vi "ReadFeatureList.vi"(8 "error in (no error)":errorcluster, 9 "Channel":string, 10 "Group":string, 11 "TDMS Ref In":refnum<k34>) -> (0 "error out":errorcluster, 1 "Channel Name Out":string, 2 "Group Name Out":string, 3 "TDMS Ref Out":refnum<k34>, 4 "Feature Display Names":string[](array[string]), 5 "Feature Code Names":string[](array[string]))   [LabVIEW 2017, in "Tdms.lvlib"]
uses:
  <vilib>/addons/InsightCM/Utilities/Tdms/Tdms.lvlib
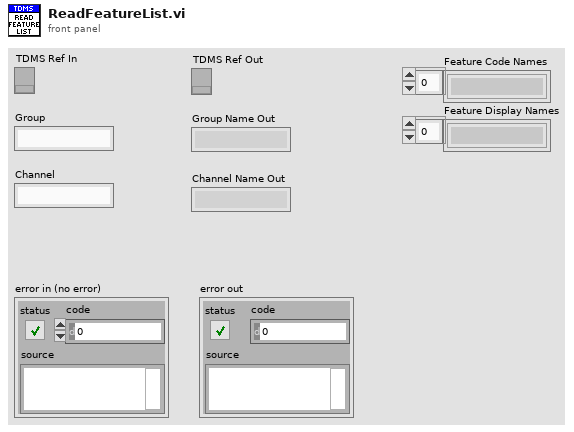
[diagram p1: front panel]
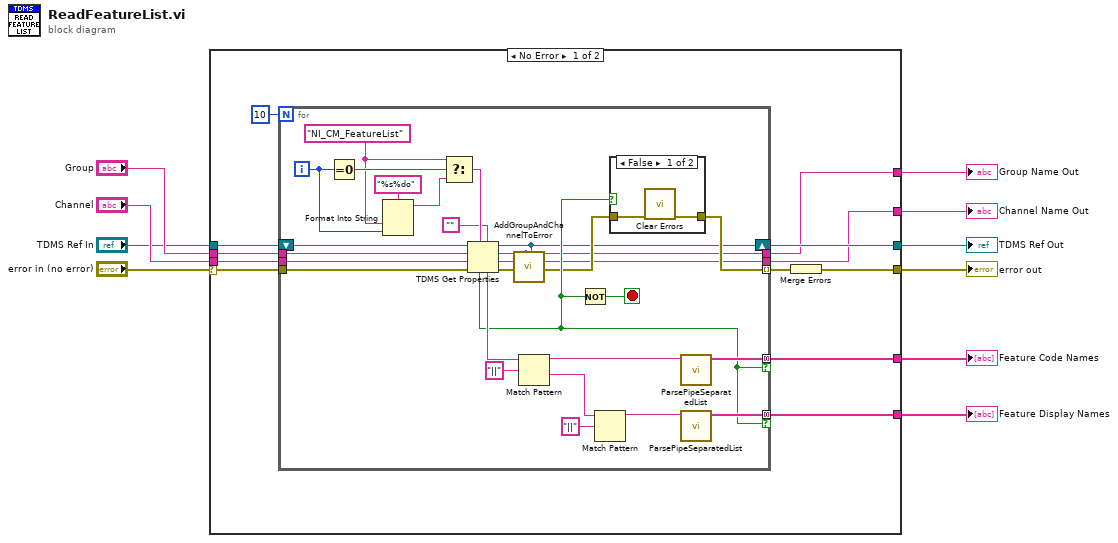
[diagram p0: block diagram]
diagram:
  n1 = case shown="No Error" "error in (no error)" {
    selector: "error in (no error)" -> [w11 w55]
    tunnel: "Group" -> [w22 w54]
    tunnel: "Channel" -> [w21 w53]
    tunnel: [w19 _] -> w8
    tunnel: [w18 _] -> w7
    tunnel: [w17 w56] -> w6
    tunnel: "TDMS Ref In" -> [w16 w56]
    tunnel: [w14 w55] -> w4
    tunnel: [w13 w54] -> w3
    tunnel: [w12 w53] -> w2
    frame No Error {
      n2 = for {
        N: 10 -> [_]
        tunnel: w22 -> [w49]
        tunnel: w11 -> [w48]
        tunnel: [w32] -> w15 mode=indexing
        tunnel: [w28] -> w12
        tunnel: [w27] -> w13
        tunnel: w21 -> [w47]
        tunnel: [w36] -> w19 mode=concatenating if=w33
        tunnel: [w35] -> w18 mode=concatenating if=w33
        shift-right: [w26] -> w17
        shift-left: w16 -> [w34]
        i -> [w41]
        stop <- w40 stop-if-true
        w42 = "NI_CM_FeatureList" ("property name")
        n3 = Equal To 0?(x=w41) -> (x = 0?=w46:bool)
        n4 = Format Into String(format string="%s%do", w42, w41) -> (resulting string=w31:string)  [unwired: 2 in, 1 out]
        n5 = Select(t=w42, s=w46, f=w31) -> (s? t:f=w45:string)
        n6 = TDMS Get Properties(5:"", 7:w45, 8:w48, 9:w47, 10:w49, 11:w34) -> (0:w30:errorcluster, 1:w28:string, 2:w27:string, 3:w26:refnum<k34>, 4:w39:string, 6:w33:bool)
        n7 = call <vilib>:"AddGroupAndChannelToError.vi"("error in (no error)"=w30, "channel name in"=w28, "group name in"=w27, "Refnum in"=w26) -> ("error out"=w29:errorcluster)  [unwired: 15 in]
        n8 = Match Pattern(string=w39, regular expression="||") -> (before substring=w37:string, after substring=w24:string)  [unwired: 1 in, 2 out]
        n9 = Not(x=w33) -> (.not. x?=w40:bool)
        n10 = Match Pattern(string=w24, regular expression="||") -> (before substring=w23:string)  [unwired: 1 in, 3 out]
        n11 = case shown="False" w33 {
          tunnel: w29 -> [w51 w52]
          tunnel: [w50 w52] -> w32
          frame False {
            n12 = call <vilib>:"Clear Errors.vi"("error in (no error)"=w51) -> ("error out"=w50:errorcluster)  [unwired: 5 in, 1 out]
          }
          frame True {
          }
        }
        n13 = call <vilib>:"ParsePipeSeparatedList.vi"("List"=w37) -> ("Array"=w36:string[])  [unwired: 10 in]
        n14 = call <vilib>:"ParsePipeSeparatedList.vi"("List"=w23) -> ("Array"=w35:string[])  [unwired: 10 in]
      }
      n15 = Merge Errors(w15) -> (w14:errorcluster)
    }
    frame Error {
    }
  }
  "error out" <- w4
  "Channel Name Out" <- w2
  "Group Name Out" <- w3
  "TDMS Ref Out" <- w6
  "Feature Code Names" <- w8
  "Feature Display Names" <- w7
